vi "Get Mouse State.vi"(8 "error in (no error)":errorcluster, 10 "Mouse":refnum<class "Mouse.lvclass">, 11 "Maze in":refnum<class "Maze.lvclass">) -> (0 "error out":errorcluster, 1 "Direction":T1, 2 "Position":T2, 3 "Maze out":refnum<class "Maze.lvclass">)   [LabVIEW 2020, in "Maze.lvlib" / "Maze.lvclass"]
uses:
  Maze.lvclass
  Mouse/Mouse.lvclass
  Position.ctl
  Direction.ctl
  Maze.lvlib
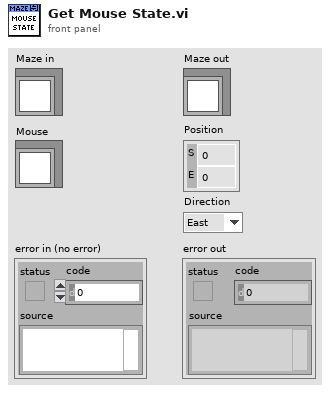
[diagram p1: front panel]
types:
  T1 = typedef "Maze.lvlib/Direction.ctl" = enum8{"East", "North", "West", "South"}
  T2 = typedef "Maze.lvlib/Position.ctl" = cluster{"S":i32, "E":i32}
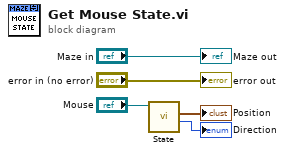
[diagram p0: block diagram]
diagram:
  n1 = call "State.vi"("Mouse in"="Mouse") -> ("Direction"=→"Direction":T1, "Position"=→"Position":T2)  [unwired: 7 in, 2 out]
  "error out" <- "error in (no error)"
  "Maze out" <- "Maze in"
